vi "wait for front panel activity.vi"() -> ()   [LabVIEW 2016]
panel:
  out "Iteration number":dbl
  out "Work done":dbl
  in  "Do some work":bool
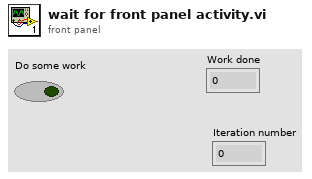
[diagram p1: front panel]
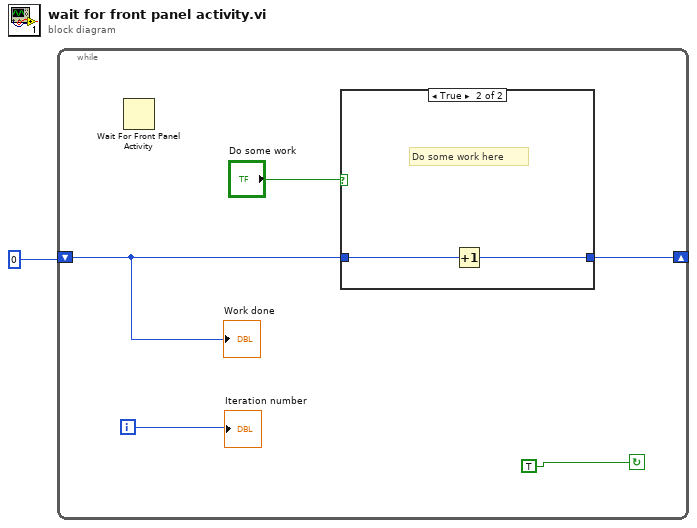
[diagram p0: block diagram]
diagram:
  n1 = while {
    shift-right: [w6] -> _
    shift-left: 0 -> [w5]
    i -> [w4]
    stop <- TRUE continue-if-true
    n2 = Wait For Front Panel Activity() -> ()  [unwired: 3 in, 1 out]
    n3 = case shown="True" "Do some work" {
      tunnel: w5 -> [_ w8]
      tunnel: [_ w7] -> w6
      frame False {
      }
      frame True {
        # "Do some work here"
        n4 = Increment(x=w8) -> (x+1=w7:i32)
      }
    }
    "Work done" <- w5
    "Iteration number" <- w4
  }
